vi "DSF.Engine.Transfer Group.Return FIFO.Write.vi"(8 "error in (no error)":errorcluster, 9 "timeout in ms (0)":i32 format="%d ms", 11 "Transfer Group in":refnum<class "DSF.Engine.Transfer Group.lvclass">) -> (0 "error out":errorcluster, 1 "timed out?":bool, 3 "Transfer Group out":refnum<class "DSF.Engine.Transfer Group.lvclass">)   [LabVIEW 2017, in "DSF.Engine.lvlib" / "DSF.Engine.Transfer Group.lvclass"]
uses:
  DSF.Engine.Transfer Group.lvclass
  DSF.Engine.Transfer Group.lvclass/DSF.Engine.Transfer Group.ctl
  Debug/DSF.Engine.Debug Flags.lvclass/DSF.Engine.Debug Flags.ctl
  Debug/DSF.Engine.Debug Flags.FIFO.lvclass/DSF.Engine.Debug Flags.FIFO.ctl
  Timing/DSF.Engine.Timing.lvclass/DSF.Engine.Timing.ctl
  Timing/DSF.Engine.Timing.lvclass
  Debug/DSF.Engine.Debug Flags.lvclass
  Debug/DSF.Engine.Debug Flags.FIFO.lvclass
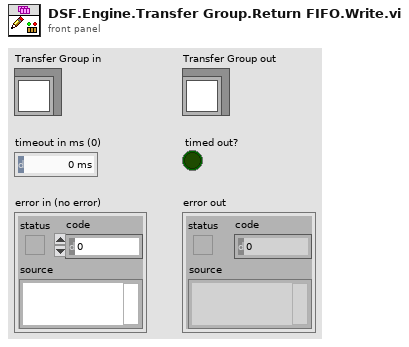
[diagram p1: front panel]
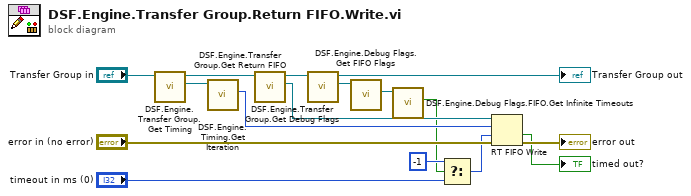
[diagram p0: block diagram]
diagram:
  n1 = call "DSF.Engine.Transfer Group.Get Timing.vi"("Transfer Group in"="Transfer Group in") -> ("Timing"=w12:refnum<class "DSF.Engine.Timing.lvclass">, "Transfer Group out"=w10:refnum<class "DSF.Engine.Transfer Group.lvclass">)  [unwired: 9 in]
  n2 = call "DSF.Engine.Timing.Get Iteration.vi"("Timing in"=w12) -> ("Iteration"=w2:u64)  [unwired: 9 in, 1 out]
  n3 = call "DSF.Engine.Transfer Group.Get Return FIFO.vi"("Transfer Group in"=w10) -> ("Return FIFO"=w16:refnum<k33>, "Transfer Group out"=w6:refnum<class "DSF.Engine.Transfer Group.lvclass">)  [unwired: 9 in]
  n4 = call "DSF.Engine.Transfer Group.Get Debug Flags.vi"("Transfer Group in"=w6) -> ("Debug Flags"=w9:refnum<class "DSF.Engine.Debug Flags.lvclass">, "Transfer Group out"=→"Transfer Group out":refnum<class "DSF.Engine.Transfer Group.lvclass">)  [unwired: 9 in]
  n5 = call "DSF.Engine.Debug Flags.Get FIFO Flags.vi"("Debug Flags in"=w9) -> ("FIFO"=w8:refnum<class "DSF.Engine.Debug Flags.FIFO.lvclass">)  [unwired: 9 in, 1 out]
  n6 = call "DSF.Engine.Debug Flags.FIFO.Get Infinite Timeouts.vi"("FIFO Debug Flags in"=w8) -> ("infinite timeouts"=w1:bool)  [unwired: 9 in, 1 out]
  n7 = Select(t=-1, s=w1, f="timeout in ms (0)") -> (s? t:f=w3:i32)
  n8 = RT FIFO Write(0:w16, 1:w2, 2:w3, 3:"error in (no error)") -> (10:→"timed out?":bool, 11:→"error out":errorcluster)  [unwired: 1 in, 2 out]
